vi "linealidad.vi"() -> ()   [LabVIEW 2010]
doc: "I. Description:\nThis example demonstrates how to take a single Measurement (Sample) from an Analog Input Channel.\n\nII. Instructions for Running:\n1. Select the Physical Channel to correspond to where your signal is input on the DAQ device.\n2. Enter the Minimum and Maximum Voltage Ranges\nNote: For better accuracy try to match the Input Ranges to the expected voltage level of the measured signal.\nNote: Use the Gen Voltage Update example to provide a signal on your DAQ device to measure.\n\nIII. Block Diagram Steps:\n1. Create an Analog Input Voltage Channel.\n2. Use the Read VI to Measure 1 Sample from 1 Channel on the Data\nAcquisition Card. Set a timeout so an error is returned if the sample\nis not returned in the specified time limit\n3. Call the Clear Task VI to clear the Task.\n4. Use the popup dialog box to display an error if any.\n\nIV. I/O Connections Overview:\nMake sure your signal input terminal matches the Physical Channel I/O Control."
uses:
  <vilib>/sound2/lvsound2.llb/Sound Data Format.ctl
  <vilib>/Utility/error.llb/DialogType.ctl
  <vilib>/sound2/lvsound2.llb/Sound Output Task ID.ctl
  <vilib>/DAQmx/read.llb/DAQmx Read (Analog DBL 1Chan 1Samp).vi
  <vilib>/DAQmx/write.llb/DAQmx Write (Analog DBL 1Chan 1Samp).vi
  <vilib>/DAQmx/create/channels.llb/DAQmx Create Channel (AI-Voltage-Basic).vi
  <vilib>/DAQmx/create/channels.llb/DAQmx Create Channel (AO-Voltage-Basic).vi
  <vilib>/Utility/file.llb/Write To Spreadsheet File (DBL).vi
  <vilib>/daqmx/miscellaneous.llb/DAQmx Fill In Error Info.vi
  <vilib>/Analysis/NI_AALBase.lvlib
panel:
  out "Vez #":i32
  out "Paso #":i32
  in  "DAC Paso":dbl step=0.001 format="%0.3f"
  in  "DAC Hasta":dbl step=0.001 format="%0.3f"
  in  "DAC Desde":dbl step=0.001 format="%0.3f"
  in  "tiempo entre pasos (ms)":dbl
  in  "Sound Paso":dbl step=0.001 format="%0.3f"
  in  "Sound Hasta":dbl step=0.001 format="%0.3f"
  in  "Sound Desde":dbl step=0.001 format="%0.3f"
  in  "DAC (T) / Sound (F)":bool
  in  "Sound Controls":T2={"device ID"=0, "sound format"={"sample rate (S/s)"=44000.0, "number of channels"=2, "bits per sample"=16}, "time (ms)"=200.0}
  out "Numeric":u32
  in  "Corre":bool
  in  "N":i32
  in  "Maximum Value 2":dbl=10.0 caption="Maximum Value" format="%.2f"
  in  "Minimum Value 2":dbl=-10.0 caption="Minimum Value" format="%0.2f"
  out "In Range?":bool
  in  "Physical Channel 2":tag="Dev1/ai0" caption="Physical Channel"
  in  "stop":bool
  in  "Maximum Value":dbl=10.0 format="%.2f"
  in  "Minimum Value":dbl=-10.0 format="%0.2f"
  in  "Physical Channel":tag="Dev1/ai0"
  # "Channel Parameters"
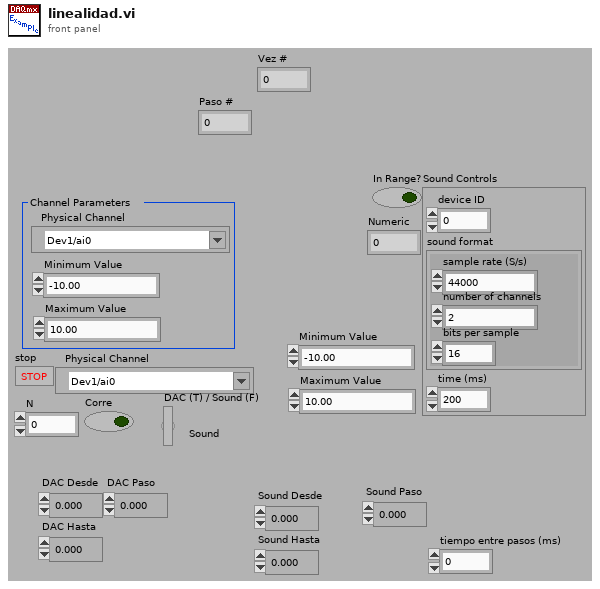
[diagram p1: front panel]
types:
  T1 = typedef "Sound Data Format.ctl" = cluster{"sample rate (S/s)":dbl, "number of channels":i32, "bits per sample":i32}
  T2 = cluster{"device ID":u32, "sound format":T1, "time (ms)":dbl}
  T3 = typedef "Sound Output Task ID.ctl" = u32
  T4 = cluster{"task ID":T3, "error":errorcluster, "sound format":T1}
  T5 = typedef "DialogType.ctl" = u16
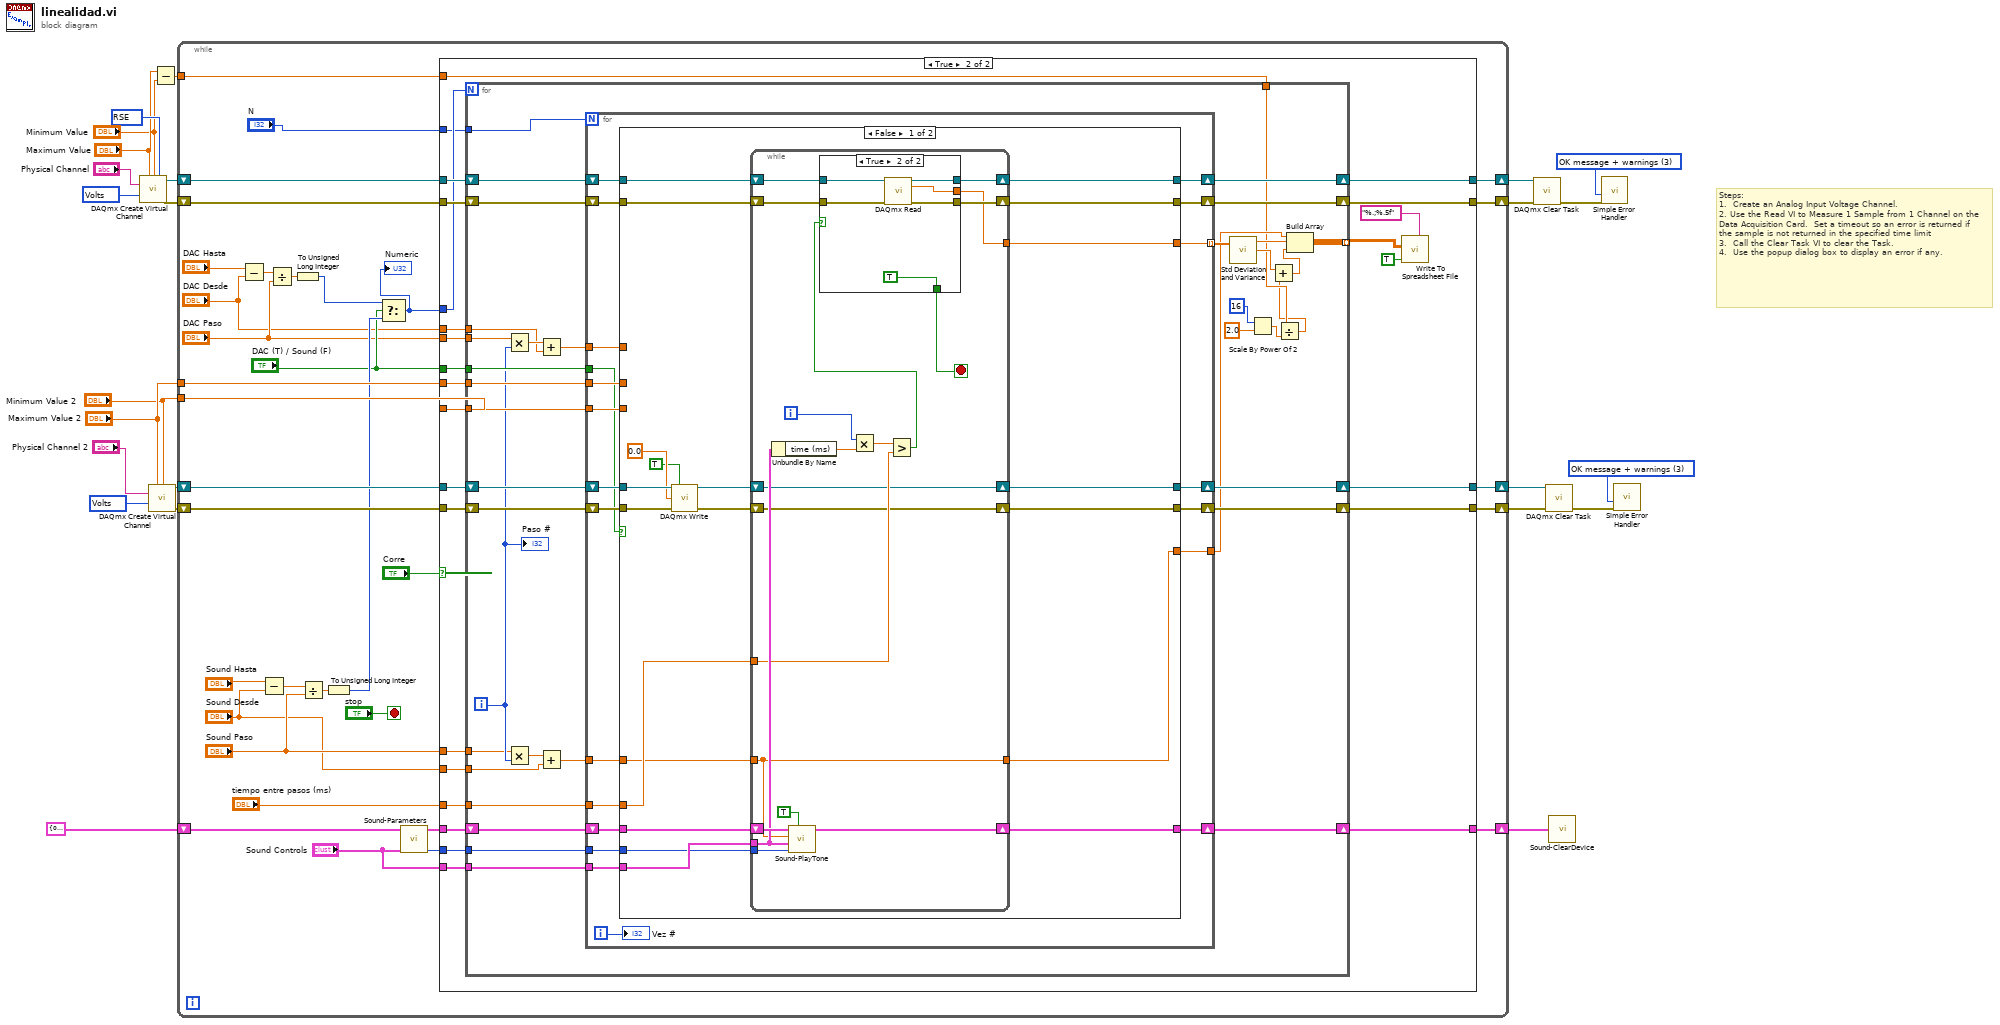
[diagram p0: block diagram]
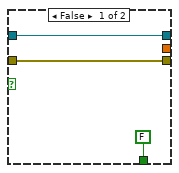
[diagram p3: hidden frame]
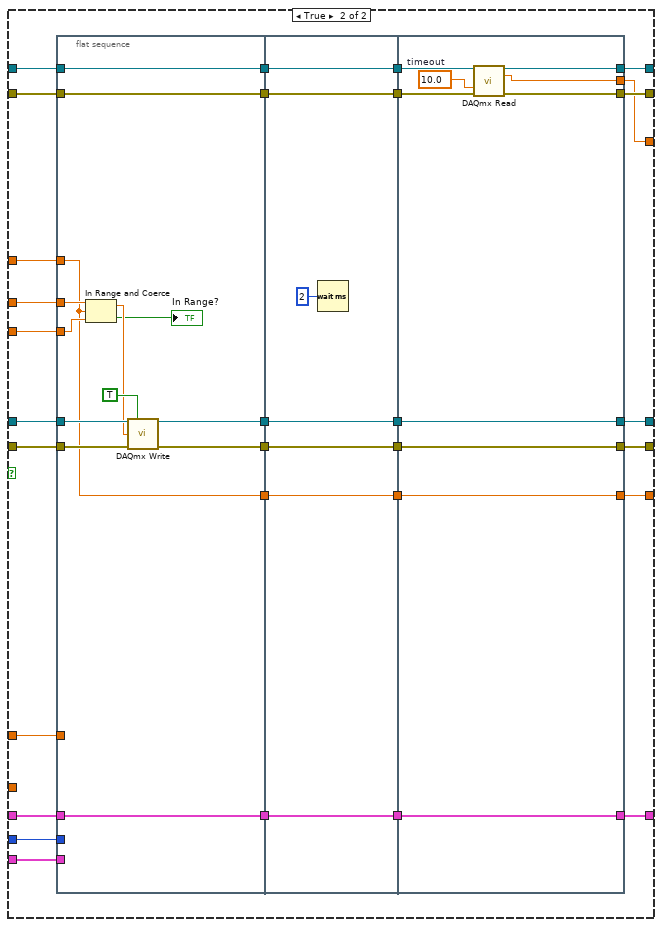
[diagram p4: hidden frame]
diagram:
  w8 = 10083 items=["default"=-1, "RSE"=10083, "NRSE"=10078, "Differential"=10106, "Pseudodifferential"=12529] ("input terminal configuration")
  w9 = 10348 items=["Volts"=10348, "From Custom Scale"=10065] ("units")
  w10 = 10348 items=["Volts"=10348, "From Custom Scale"=10065] ("units")
  w14 = T5 3 items=["no dialog", "OK message", "continue or stop message", "OK message + warnings", "continue/stop + warnings"] ("type of dialog (OK msg:1)")
  w21 = T5 3 items=["no dialog", "OK message", "continue or stop message", "OK message + warnings", "continue/stop + warnings"] ("type of dialog (OK msg:1)")
  # "Steps: \n1.  Create an Analog Input Voltage Channel. \n2. Use the Read VI to Measure 1 Sample from 1 Channel on the Data Acquisition Card.  Set a timeout so an error is returned if the sample is not returned in the specified time limit\n3.  Call the Clear Task VI to clear the Task.\n4.  Use the popup dialog box to display an error if any."
  n1 = call-poly <vilib>:"DAQmx Create Virtual Channel.vi"("maximum value"="Maximum Value", "minimum value"="Minimum Value", "input terminal configuration"=w8, "physical channels"="Physical Channel", "units"=w10) -> ("task out"=w23:refnum<k21>, "error out"=w22:errorcluster)  [unwired: 9 in]
  n2 = call-poly <vilib>:"DAQmx Create Virtual Channel.vi"("maximum value"="Maximum Value 2", "minimum value"="Minimum Value 2", "physical channels"="Physical Channel 2", "units"=w9) -> ("task out"=w16:refnum<k21>, "error out"=w15:errorcluster)  [unwired: 10 in]
  n3 = Subtract(x="Maximum Value", y="Minimum Value") -> (x-y=w1:dbl)
  n4 = while {
    shift-right: [w52] -> w20
    shift-left: w23 -> [w55]
    shift-right: [w53] -> w19
    shift-left: w22 -> [w54]
    shift-right: [w51] -> w12
    shift-left: w16 -> [w57]
    shift-right: [w50] -> w11
    shift-left: w15 -> [w56]
    tunnel: "Maximum Value 2" -> [w49]
    tunnel: "Minimum Value 2" -> [w48]
    shift-right: [w44] -> w4
    shift-left: T4 {"task ID"=0, "error"={"status"=TRUE, "code"=0, "source"=""}, "sound format"={"sample rate (S/s)"=0.0, "number of channels"=0, "bits per sample"=0}} ("Sound Device OUT") -> [w46]
    tunnel: w1 -> [w25]
    stop <- "stop" stop-if-true
    n5 = Subtract(x="DAC Hasta", y="DAC Desde") -> (x-y=w31:dbl)
    n6 = Subtract(x="Sound Hasta", y="Sound Desde") -> (x-y=w40:dbl)
    n7 = Divide(x=w31, y="DAC Paso") -> (x/y=w30:dbl)
    n8 = To Unsigned Long Integer(number=w30) -> (unsigned 32bit integer=w29:u32)
    n9 = Divide(x=w40, y="Sound Paso") -> (x/y=w39:dbl)
    n10 = To Unsigned Long Integer(number=w39) -> (unsigned 32bit integer=w34:u32)
    n11 = Select(t=w29, s="DAC (T) / Sound (F)", f=w34) -> (s? t:f=w41:u32)
    "Numeric" <- w41
    n12 = call "Sound-Parameters.vi"("Sound Controls"="Sound Controls", "Sound Device IN"=w46) -> ("#samples"=w43:u32, "Sound Device OUT"=w45:T4)  [unwired: 3 in, 1 out]
    n13 = case shown="True" "Corre" {
      tunnel: w57 -> [w61 w89]
      tunnel: w56 -> [w60 w88]
      tunnel: w55 -> [w63 w87]
      tunnel: w54 -> [w62 w86]
      tunnel: [w62 w85] -> w53
      tunnel: [w63 w84] -> w52
      tunnel: [w61 w83] -> w51
      tunnel: [w60 w82] -> w50
      tunnel: w49 -> [_ w81]
      tunnel: w48 -> [_ w80]
      tunnel: w41 -> [_ w79]
      tunnel: "DAC Paso" -> [_ w78]
      tunnel: "DAC Desde" -> [_ w77]
      tunnel: "N" -> [_ w76]
      tunnel: "DAC (T) / Sound (F)" -> [_ w72]
      tunnel: w45 -> [w59 w71]
      tunnel: [w59 w70] -> w44
      tunnel: w43 -> [_ w69]
      tunnel: "Sound Controls" -> [_ w68]
      tunnel: "Sound Paso" -> [_ w67]
      tunnel: "Sound Desde" -> [_ w66]
      tunnel: "tiempo entre pasos (ms)" -> [_ w65]
      tunnel: w25 -> [_ w64]
      frame False {
      }
      frame True {
        n14 = for {
          N: w79 -> [_]
          tunnel: w81 -> [w118]
          tunnel: w80 -> [w117]
          shift-right: [w122] -> w85
          shift-left: w86 -> [w123]
          shift-right: [w121] -> w84
          shift-left: w87 -> [w124]
          shift-right: [w120] -> w83
          shift-left: w89 -> [w126]
          shift-right: [w119] -> w82
          shift-left: w88 -> [w125]
          tunnel: w78 -> [w115]
          tunnel: w77 -> [w114]
          tunnel: w76 -> [w113]
          tunnel: [w111] -> w75 mode=indexing
          tunnel: w72 -> [w107]
          shift-right: [w105] -> w70
          shift-left: w71 -> [w106]
          tunnel: w69 -> [w104]
          tunnel: w68 -> [w103]
          tunnel: w67 -> [w100]
          tunnel: w66 -> [w99]
          tunnel: w65 -> [w97]
          tunnel: w64 -> [w92]
          i -> [w101]
          n15 = Multiply(x=w115, y=w101) -> (x*y=w116:dbl)
          n16 = Multiply(x=w100, y=w101) -> (x*y=w102:dbl)
          n17 = Add(x=w116, y=w114) -> (x+y=w109:dbl)
          n18 = Add(x=w102, y=w99) -> (x+y=w98:dbl)
          n19 = for {
            N: w113 -> [_]
            tunnel: w118 -> [w139]
            tunnel: w117 -> [w138]
            shift-right: [w142] -> w121
            shift-left: w124 -> [w145]
            shift-right: [w143] -> w122
            shift-left: w123 -> [w144]
            shift-right: [w141] -> w120
            shift-left: w126 -> [w147]
            shift-right: [w140] -> w119
            shift-left: w125 -> [w146]
            tunnel: w109 -> [w137]
            tunnel: [w136] -> w110 mode=indexing
            tunnel: [w135] -> w108
            tunnel: w107 -> [w128]
            shift-right: [w133] -> w105
            shift-left: w106 -> [w134]
            tunnel: w104 -> [w132]
            tunnel: w103 -> [w131]
            tunnel: w98 -> [w130]
            tunnel: w97 -> [w129]
            i -> [w127]
            n20 = case shown="False" w128 {
              tunnel: w147 -> [w150 w213]
              tunnel: w146 -> [w151 w212]
              tunnel: w145 -> [w165 w211]
              tunnel: w144 -> [w163 w210]
              tunnel: [w162 w209] -> w143
              tunnel: [w164 w208] -> w142
              tunnel: [w155 w207] -> w141
              tunnel: [w156 w206] -> w140
              tunnel: w139 -> [_ w205]
              tunnel: w138 -> [_ w204]
              tunnel: w137 -> [_ w203]
              tunnel: [w157 w202] -> w136
              tunnel: [w154 w201] -> w135
              tunnel: w134 -> [w167 w200]
              tunnel: [w166 w199] -> w133
              tunnel: w132 -> [w160 w198]
              tunnel: w131 -> [w161 w197]
              tunnel: w130 -> [w158 w196]
              tunnel: w129 -> [w159 _]
              frame False {
                n21 = call-poly <vilib>:"DAQmx Write.vi"("task/channels in"=w150, "auto start"=TRUE, "data"=0.0, "error in"=w151) -> ("task out"=w153:refnum<k21>, "error out"=w152:errorcluster)  [unwired: 9 in, 1 out]
                n22 = while {
                  tunnel: w159 -> [w178]
                  tunnel: w158 -> [w168]
                  tunnel: w161 -> [w180]
                  tunnel: w160 -> [w182]
                  shift-right: [w183] -> w164
                  shift-left: w165 -> [w184]
                  shift-right: [w185] -> w166
                  shift-left: w167 -> [w186]
                  shift-right: [w175] -> w162
                  shift-left: w163 -> [w174]
                  tunnel: [w173] -> w157
                  shift-right: [w171] -> w155
                  shift-left: w153 -> [w171]
                  shift-right: [w172] -> w156
                  shift-left: w152 -> [w172]
                  tunnel: [w168] -> w154
                  i -> [w169]
                  stop <- w177 stop-if-true
                  n23 = Unbundle By Name(w180) -> ("time (ms)"=w170:dbl)
                  n24 = call "Sound-PlayTone.vi"("sound?"=TRUE ("DAQ?"), "# samples"=w182, "Sound Controls"=w180, "Frecuencia"=w168, "Sound Device IN"=w186) -> ("Sound Device OUT"=w185:T4)  [unwired: 3 in, 1 out]
                  n25 = Multiply(x=w169, y=w170) -> (x*y=w179:dbl)
                  n26 = Greater?(x=w179, y=w178) -> (0:w176:bool)
                  n27 = case shown="True" w176 {
                    tunnel: w184 -> [w189 w195]
                    tunnel: [w189 w194] -> w183
                    tunnel: [FALSE ("Streeam") TRUE ("Streeam")] -> w177
                    tunnel: [w187 w192] -> w175
                    tunnel: w174 -> [w187 w191]
                    tunnel: [_ w190] -> w173
                    frame False {
                    }
                    frame True {
                      n28 = call-poly <vilib>:"DAQmx Read.vi"("task/channels in"=w195, "error in"=w191) -> ("task out"=w194:refnum<k21>, "data"=w190:dbl, "error out"=w192:errorcluster)  [unwired: 11 in]
                    }
                  }
                }
              }
              frame True {
                n29 = flat-sequence {
                  tunnel: w213 -> [w236]
                  tunnel: w212 -> [w235]
                  tunnel: [w238] -> w225
                  tunnel: w211 -> [w238]
                  tunnel: w210 -> [w237]
                  tunnel: [w237] -> w224
                  tunnel: [w234] -> w223
                  tunnel: [w233] -> w222
                  tunnel: w205 -> [w232]
                  tunnel: w204 -> [w231]
                  tunnel: w203 -> [w230]
                  tunnel: [w230] -> w221
                  tunnel: w200 -> [w229]
                  tunnel: [w229] -> w220
                  tunnel: w198 -> [_]
                  tunnel: w197 -> [_]
                  tunnel: w196 -> [_]
                  tunnel: w225 -> [w245]
                  tunnel: [w245] -> w219
                  tunnel: w224 -> [w244]
                  tunnel: [w244] -> w218
                  tunnel: w223 -> [w243]
                  tunnel: [w243] -> w217
                  tunnel: w222 -> [w242]
                  tunnel: [w242] -> w216
                  tunnel: w221 -> [w241]
                  tunnel: [w241] -> w215
                  tunnel: [w240] -> w214
                  tunnel: w220 -> [w240]
                  tunnel: w219 -> [w254]
                  tunnel: w218 -> [w253]
                  tunnel: [w252] -> w209
                  tunnel: [w251] -> w208
                  tunnel: w217 -> [w250]
                  tunnel: [w250] -> w207
                  tunnel: w216 -> [w249]
                  tunnel: [w249] -> w206
                  tunnel: [w248] -> w202
                  tunnel: w215 -> [w247]
                  tunnel: [w247] -> w201
                  tunnel: [w246] -> w199
                  tunnel: w214 -> [w246]
                  frame #0 {
                    n30 = In Range and Coerce(upper limit=w232, x=w230, lower limit=w231) -> (coerced(x)=w227:dbl, In Range?=→"In Range?":bool)
                    n31 = call-poly <vilib>:"DAQmx Write.vi"("task/channels in"=w236, "auto start"=TRUE, "data"=w227, "error in"=w235) -> ("task out"=w234:refnum<k21>, "error out"=w233:errorcluster)  [unwired: 9 in, 1 out]
                  }
                  frame #1 {
                    n32 = Wait (ms)(milliseconds to wait=u32 2) -> ()  [unwired: 1 out]
                  }
                  frame #2 {
                    w255 = 10.0  # timeout
                    n33 = call-poly <vilib>:"DAQmx Read.vi"("task/channels in"=w254, "timeout"=w255, "error in"=w253) -> ("task out"=w251:refnum<k21>, "data"=w248:dbl, "error out"=w252:errorcluster)  [unwired: 10 in]
                  }
                }
              }
            }
            "Vez #" <- w127
          }
          n34 = call <vilib>:"Std Deviation and Variance.vi"("X"=w110) -> ("mean"=w112:dbl, "standard deviation"=w96:dbl)  [unwired: 1 in, 1 out]
          n35 = Scale By Power Of 2(n=16, x=2.0) -> (x*2^n=w91:dbl)
          n36 = Divide(x=w92, y=w91) -> (x/y=w90:dbl)
          n37 = Add(x=w96, y=w90) -> (x+y=w95:dbl)
          n38 = Build Array(w108, w112, w95) -> (w111:dbl[])
          "Paso #" <- w101
        }
        n39 = call-poly <vilib>:"Write To Spreadsheet File.vi"("format (%.3f)"="%.;%.5f", "append to file? (new file:F)"=TRUE, "2D data"=w75) -> ()  [unwired: 5 in, 1 out]
      }
    }
  }
  n40 = call <vilib>:"DAQmx Clear Task.vi"("task in"=w20, "error in"=w19) -> ("error out"=w18:errorcluster)  [unwired: 13 in]
  n41 = call <vilib>:"DAQmx Clear Task.vi"("task in"=w12, "error in"=w11) -> ("error out"=w13:errorcluster)  [unwired: 13 in]
  n42 = call "Sound-ClearDevice.vi"("Sound Device OUT"=w4) -> ()
  n43 = call <vilib>:"Simple Error Handler.vi"("type of dialog (OK msg:1)"=w21, "error in (no error)"=w18) -> ()  [unwired: 3 in, 5 out]
  n44 = call <vilib>:"Simple Error Handler.vi"("type of dialog (OK msg:1)"=w14, "error in (no error)"=w13) -> ()  [unwired: 3 in, 5 out]
